vi "FGV Rohmesswerte sammeln.vi"(0 "Rohwerte":sgl[](array[numeric]), 5 "MFC in":u32, 7 "Sollwert":dbl, 11 "error in (no error)":errorcluster caption="Fehler (Eingang, kein Fehler)", 13 "Aktion":T2) -> (4 "Rohmessdaten":sgl[][](array[numeric]), 8 "Sollwert je MFC Cluster":T1, 10 "Aktueller Sollwert je MFC":dbl[](array[numeric]), 15 "error out":errorcluster caption="Fehler (Ausgang)")   [LabVIEW 2020, in "Linearisierung v2.lvlib"]
uses:
  Linearisierung v2.lvlib
  Aktion FGV Rohmesswerte sammeln.ctl
  HovaCAL Sollwerte je MFC Cluster.ctl
  Seiten/EL3000/Allgemeine VI/Aktion FGV Werte Standardanalysator.ctl
  Messdaten/Messdaten.lvlib
  Seiten/EL3000/Allgemeine VI/Allgemeine VI.lvlib
  Gasteiler/HovaCAL_Interface/Kommunikation/Kommunikation.lvlib
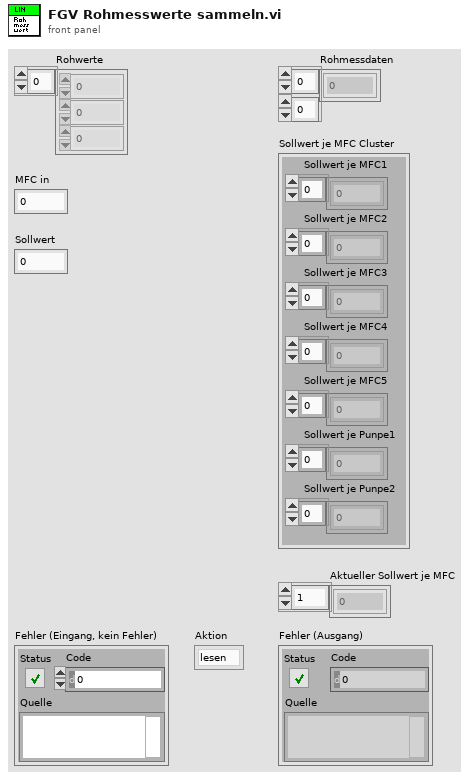
[diagram p1: front panel]
types:
  T1 = typedef "Linearisierung v2.lvlib/HovaCAL Sollwerte je MFC Cluster.ctl" = cluster{"Sollwert je MFC1":sgl[], "Sollwert je MFC2":sgl[], "Sollwert je MFC3":sgl[], "Sollwert je MFC4":sgl[], "Sollwert je MFC5":sgl[], "Sollwert je Punpe1":sgl[], "Sollwert je Punpe2":sgl[]}
  T2 = typedef "Linearisierung v2.lvlib/Aktion FGV Rohmesswerte sammeln.ctl" = enum16{"lesen", "schreiben", "löschen", "Sollwert HovaCal"}
  T3 = typedef "ABB-EL3000.lvlib/Allgemeine VI.lvlib/Aktion FGV Werte Standardanalysator.ctl" = enum16{"lesen", "FID", "PMA"}
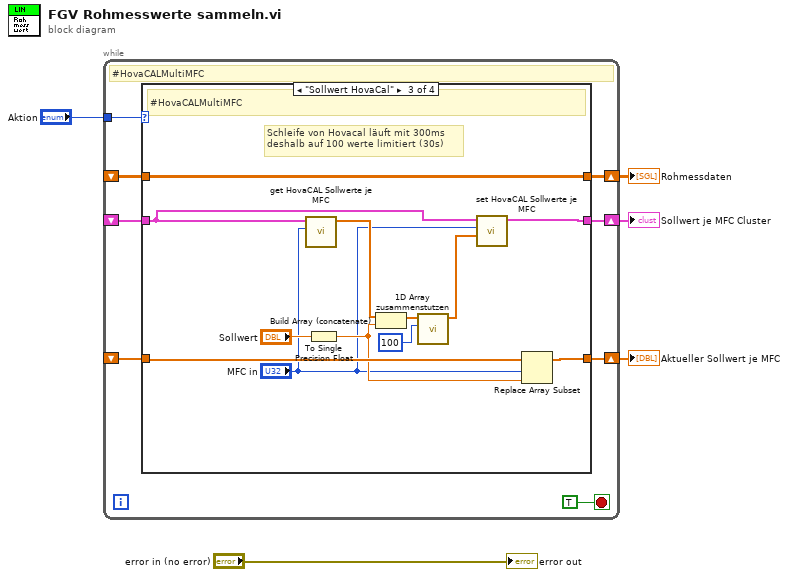
[diagram p0: block diagram]
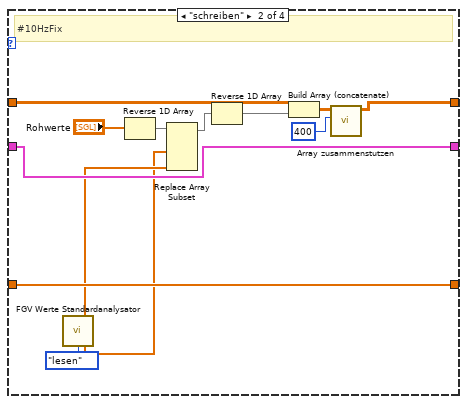
[diagram p3: hidden frame]
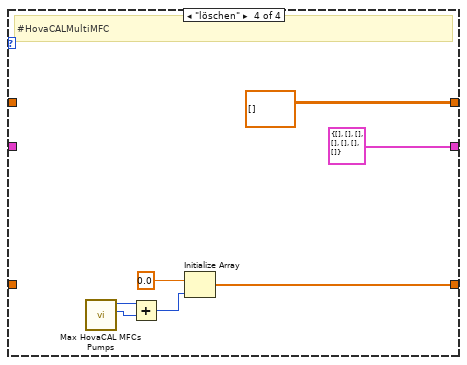
[diagram p4: hidden frame]
diagram:
  n1 = while {
    tunnel: "Aktion" -> [w12]
    shift-right: [w11] -> w4
    shift-left: _ -> [w10]
    shift-right: [w9] -> w1
    shift-left: _ -> [w8]
    shift-right: [w7] -> w3
    shift-left: _ -> [w6]
    stop <- TRUE stop-if-true
    # "#HovaCALMultiMFC"
    n2 = case shown="\"Sollwert HovaCal\"" w12 {
      tunnel: [w16 w26 w41 sgl[][] []] -> w11
      tunnel: w10 -> [w16 w27 w41 _]
      tunnel: [w15 w25 w30 T1 {"Sollwert je MFC1"=[], "Sollwert je MFC2"=[], "Sollwert je MFC3"=[], "Sollwert je MFC4"=[], "Sollwert je MFC5"=[], "Sollwert je Punpe1"=[], "Sollwert je Punpe2"=[]} ("Sollwert je MFC Cluster")] -> w9
      tunnel: w8 -> [w15 w25 w34 _]
      tunnel: [w14 w24 w37 w43] -> w7
      tunnel: w6 -> [w14 w24 w38 _]
      frame "lesen", Default {
      }
      frame "schreiben" {
        # "#10HzFix"
        n3 = call "FGV Werte Standardanalysator.vi"("Aktion"=Aktion_FGV_Werte_Standardanalysator."lesen") -> ("FID Rohwerte LIN"=w20:sgl[], "PMA Rohwerte LIN"=w17:sgl[])  [unwired: 8 in, 5 out]
        n4 = Reverse 1D Array(array="Rohwerte") -> (reversed array=w21:sgl[])
        n5 = Replace Array Subset(array=w21, new element #1=w17, new element #2=w20) -> (w19:sgl[])  [unwired: 2 in]
        n6 = Reverse 1D Array(array=w19) -> (reversed array=w18:sgl[])
        n7 = Build Array (concatenate)(w27, w18) -> (w29:sgl[][])
        n8 = call "Array zusammenstutzen.vi"("Anzahl Elemente"=400, "Messdaten"=w29) -> ("Messdaten"=w26:sgl[][])  [unwired: 8 in, 1 out]
      }
      frame "Sollwert HovaCal" {
        # "Schleife von Hovacal läuft mit 300ms\ndeshalb auf 100 werte limitiert (30s)"
        # "#HovaCALMultiMFC"
        n9 = call "get HovaCAL Sollwerte je MFC.vi"("MFC in"="MFC in", "Sollwert je MFC Cluster"=w34) -> ("Sollwert MFC"=w35:sgl[])  [unwired: 9 in]
        n10 = To Single Precision Float(number="Sollwert") -> (single precision float=w32:sgl)
        n11 = Build Array (concatenate)(w35, w32) -> (w40:sgl[])
        n12 = call "1D Array zusammenstutzen.vi"("Anzahl Elemente"=100, "Messdaten"=w40) -> ("Messdaten"=w33:sgl[])  [unwired: 8 in, 1 out]
        n13 = call "set HovaCAL Sollwerte je MFC.vi"("Messdaten"=w33, "MFC in"="MFC in", "Sollwert je MFC Cluster (Eingang)"=w34) -> ("Sollwert je MFC Cluster (Ausgang)"=w30:T1)  [unwired: 8 in]
        n14 = Replace Array Subset(array=w38, new element=w32, index="MFC in") -> (w37:dbl[])
      }
      frame "löschen" {
        # "#HovaCALMultiMFC"
        n15 = call "Max HovaCAL MFCs Pumps.vi"() -> ("max Pumps"=w46:i32, "max MFCs"=w47:i32)  [unwired: 10 in]
        n16 = Add(x=w47, y=w46) -> (x+y=w45:i32)
        n17 = Initialize Array(0.0 ("Sollwert"), w45) -> (w43:dbl[])
      }
    }
  }
  "Rohmessdaten" <- w4
  "Aktueller Sollwert je MFC" <- w3
  "Sollwert je MFC Cluster" <- w1
  "error out" <- "error in (no error)"
